vi "In_Range_check.vi"(1 "±":dbl format="%.2f", 4 "%":dbl format="%.2f", 5 "Mode":T1, 6 "Value":dbl format="%.2f", 7 "Setpoint":dbl format="%.2f") -> (2 "In Range":bool)   [LabVIEW 2010]
uses:
  Controls/In_Range.ctl
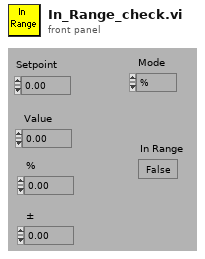
[diagram p1: front panel]
types:
  T1 = typedef "In_Range.ctl" = enum16{"%", "±", "% & ±"}
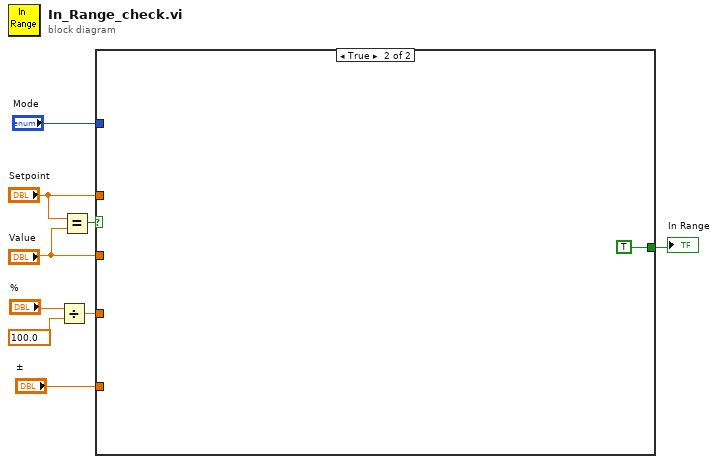
[diagram p0: block diagram]
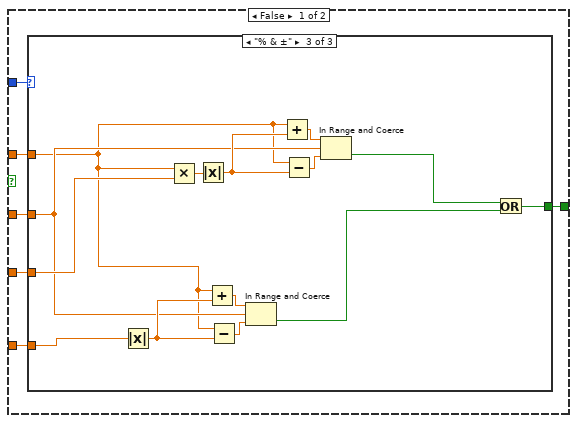
[diagram p2: hidden frame]
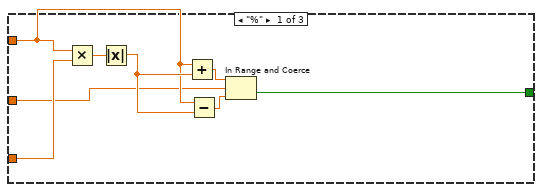
[diagram p3: hidden frame]
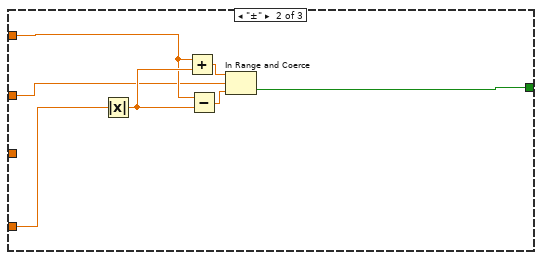
[diagram p4: hidden frame]
diagram:
  n1 = Divide(x="%", y=100.0) -> (x/y=w6:dbl)
  n2 = Equal?(x="Setpoint", y="Value") -> (x = y?=w1:bool)
  n3 = case shown="True" w1 {
    tunnel: "Mode" -> [w15 _]
    tunnel: "Setpoint" -> [w14 _]
    tunnel: w6 -> [w13 _]
    tunnel: "Value" -> [w12 _]
    tunnel: [w11 TRUE] -> w5
    tunnel: "±" -> [w10 _]
    frame False {
      n4 = case shown="\"% & ±\"" w15 {
        tunnel: w14 -> [w18 w27 w34]
        tunnel: w13 -> [w23 _ w37]
        tunnel: w12 -> [w17 w26 w35]
        tunnel: [w16 w24 w31] -> w11
        tunnel: w10 -> [_ w25 w41]
        frame "%" {
          n5 = Multiply(x=w18, y=w23) -> (x*y=w22:dbl)
          n6 = Absolute Value(x=w22) -> (abs(x)=w21:dbl)
          n7 = Add(x=w18, y=w21) -> (x+y=w19:dbl)
          n8 = Subtract(x=w18, y=w21) -> (x-y=w20:dbl)
          n9 = In Range and Coerce(upper limit=w19, x=w17, lower limit=w20) -> (In Range?=w16:bool)  [unwired: 1 out]
        }
        frame "±" {
          n10 = Absolute Value(x=w25) -> (abs(x)=w30:dbl)
          n11 = Add(x=w27, y=w30) -> (x+y=w28:dbl)
          n12 = Subtract(x=w27, y=w30) -> (x-y=w29:dbl)
          n13 = In Range and Coerce(upper limit=w28, x=w26, lower limit=w29) -> (In Range?=w24:bool)  [unwired: 1 out]
        }
        frame "% & ±" {
          n14 = Absolute Value(x=w41) -> (abs(x)=w44:dbl)
          n15 = Multiply(x=w34, y=w37) -> (x*y=w36:dbl)
          n16 = Absolute Value(x=w36) -> (abs(x)=w38:dbl)
          n17 = Add(x=w34, y=w44) -> (x+y=w42:dbl)
          n18 = Subtract(x=w34, y=w44) -> (x-y=w43:dbl)
          n19 = In Range and Coerce(upper limit=w42, x=w35, lower limit=w43) -> (In Range?=w32:bool)  [unwired: 1 out]
          n20 = Add(x=w34, y=w38) -> (x+y=w40:dbl)
          n21 = Subtract(x=w34, y=w38) -> (x-y=w39:dbl)
          n22 = In Range and Coerce(upper limit=w40, x=w35, lower limit=w39) -> (In Range?=w33:bool)  [unwired: 1 out]
          n23 = Or(x=w33, y=w32) -> (x .or. y?=w31:bool)
        }
      }
    }
    frame True {
    }
  }
  "In Range" <- w5
